vi "Destroy.vi"(8 "error in (no error)":errorcluster, 11 "Map in":refnum<class "ObjectMap.lvclass">) -> (0 "error out":errorcluster, 5 "MapImp out":refnum<class "MapImp.lvclass">, 7 "Map out":refnum<class "ObjectMap.lvclass">)   [LabVIEW 2013, in "LapDog.Collections.v1.Maps.lvlib" / "ObjectMap.lvclass"]
doc: "Add a key-value pair to the map.\n\nIf the key already exists, error 510202 is returned."
uses:
  ObjectMap.lvclass
  MapImp/MapImp.lvclass
  ObjectMap.lvclass/ObjectMap.ctl
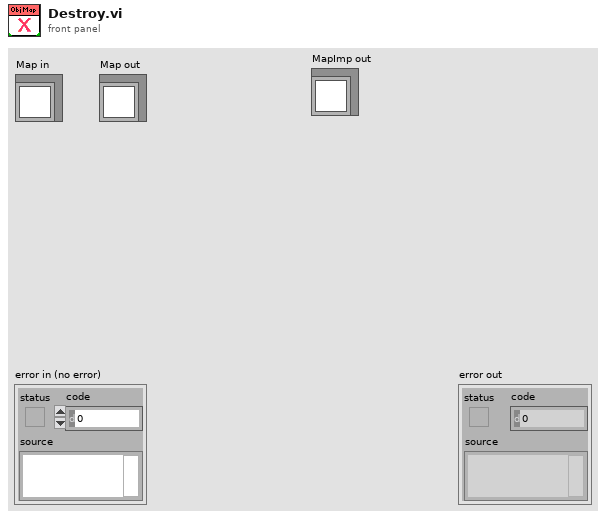
[diagram p1: front panel]
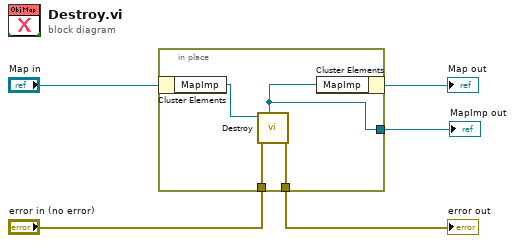
[diagram p0: block diagram]
diagram:
  n1 = in-place {
    in-place-border: "error in (no error)" -> [w8]
    in-place-border: [w7] -> w2
    in-place-border: [w6] -> w1
    n2 = in-place-cluster #1("Map in") -> ("MapImp"=w9:refnum<class "MapImp.lvclass">)
    n3 = call-dynamic "Destroy.vi"("error in (no error)"=w8, "VariantAttribute in"=w9) -> ("error out"=w7:errorcluster, "VariantAttribute out"=w6:refnum<class "MapImp.lvclass">)  [unwired: 8 in]
    n4 = in-place-cluster #1("MapImp"=w6) -> (→"Map out":refnum<class "ObjectMap.lvclass">)
  }
  "error out" <- w2
  "MapImp out" <- w1
